vi "Export JUnit.vi"(8 "error in (no error)":errorcluster) -> (0 "error out":errorcluster)   [LabVIEW 2013, in "Test Runner.JUnit.lvclass"]
uses:
  Test Runner.JUnit.lvclass
  classes/Assert/Assert Greater Or Equal_Variant.vi
  classes/Test/Test.lvclass
  classes/Assert/Assert.lvclass
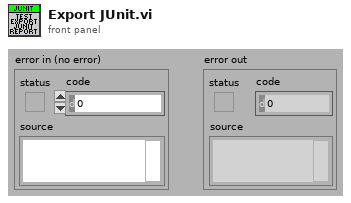
[diagram p1: front panel]
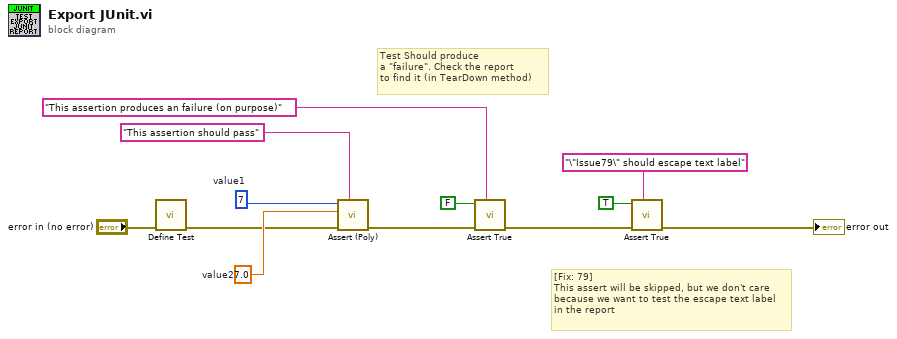
[diagram p0: block diagram]
diagram:
  w9 = 7.0  # value2
  w10 = 7  # value1
  # "[Fix: 79] \nThis assert will be skipped, but we don't care\nbecause we want to test the escape text label\nin the report"
  # "Test Should produce\na \"failure\". Check the report\nto find it (in TearDown method)"
  n1 = call "Define Test.vi"("error in (no error)"="error in (no error)") -> ("error out"=w8:errorcluster)  [unwired: 10 in]
  n2 = call-poly "Assert (Poly).vi"("Label"="This assertion should pass", "error in (no error)"=w8, "Y"=w9, "X"=w10) -> ("error out"=w7:errorcluster)  [unwired: 7 in]
  n3 = call "Assert True.vi"("Label"="This assertion produces an failure (on purpose)", "error in (no error)"=w7, "True?"=FALSE) -> ("error out"=w3:errorcluster)  [unwired: 8 in]
  n4 = call "Assert True.vi"("Label"="\"Issue79\" should escape text label", "error in (no error)"=w3, "True?"=TRUE) -> ("error out"=→"error out":errorcluster)  [unwired: 8 in]
